vi "TriggerTests_2b_long.vi"() -> ()   [LabVIEW 2009]
uses:
  <vilib>/Utility/NIReport.llb/NI_report.lvclass
panel:
  in  "Instrument VISA in":T1={"AWG VISA"="81160A", "Oscilloscope  VISA "="DSO80204B", "Integration Board IP"="172.16.7.43", "connection ID"=refnum, "report out"=refnum, "report file path"=path "D:/CTA/LevelTriggerBoardTest/TestsData/sumtrigger_delay/dataruben"}
  in  "test 2.3a":bool=TRUE
  in  "report file path":path=path "D:/CTA/LevelTriggerBoardTest/TestsData/sumtrigger_delay/dataruben/report.htm"
  out "error out":errorcluster
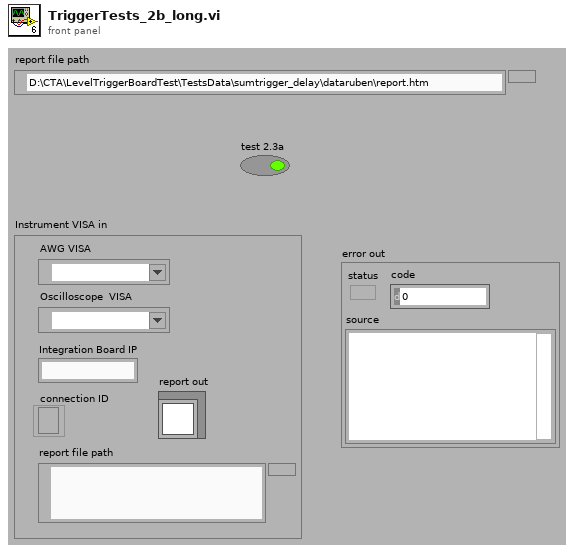
[diagram p1: front panel]
types:
  T1 = cluster{"AWG VISA":refnum<visa-resource-name>, "Oscilloscope  VISA ":refnum<visa-resource-name>, "Integration Board IP":string, "connection ID":refnum<k5>, "report out":refnum<class "NI_report.lvclass">, "report file path":path}
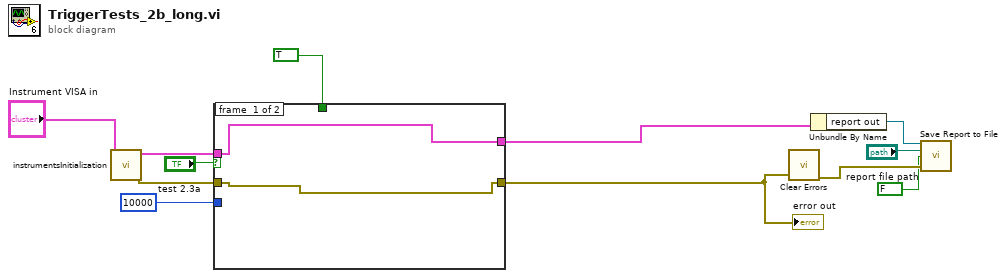
[diagram p0: block diagram]
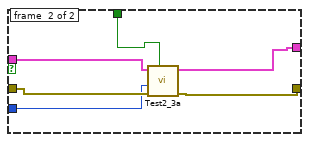
[diagram p2: hidden frame]
diagram:
  n1 = call "instrumentsInitialization.vi"("Instrument VISA in"="Instrument VISA in") -> ("error out"=w6:errorcluster, "Instrument VISA out"=w12:T1)  [unwired: 9 in]
  n2 = case shown="True" "test 2.3a" {
    tunnel: w6 -> [w13 w20]
    tunnel: w12 -> [w14 w15]
    tunnel: 10000 ("Cycles Burst") -> [_ w17]
    tunnel: [w13 w19] -> w5
    tunnel: [w14 w16] -> w4
    tunnel: TRUE ("Report Enable") -> [_ w18]
    frame #0 {
    }
    frame #1 {
      n3 = call "Test2_3a.vi"("Report Enable"=w18, "error in"=w20, "Cycles Burst"=w17, "Instrument VISA in"=w15) -> ("error out"=w19:errorcluster, "Instrument VISA out"=w16:T1)  [unwired: 6 in]
    }
  }
  "error out" <- w5
  n4 = call <vilib>:"Clear Errors.vi"("error in (no error)"=w5) -> ("error out"=w8:errorcluster)  [unwired: 6 in]
  n5 = Unbundle By Name(w4) -> ("report out"=w11:refnum<class "NI_report.lvclass">)
  n6 = call-dynamic "Save Report to File.vi"("report in"=w11, "report file path"="report file path", "prompt to replace? (F)"=FALSE, "error in (no error)"=w8) -> ()  [unwired: 10 in, 2 out]
